vi "_TangoGroupWriteAttribute.vi"(1 "error in":errorcluster, 2 "values":T1(array[cluster]), 3 "attribute name":string, 4 "group id":i32) -> (0 "error out":errorcluster)   [LabVIEW 2014, in "tango.lvlib"]
uses:
  tango.lvlib
  tango_binding.so
panel:
  # "*** READ-ME ***\n\nThis Vi can only write one atrribute at a time on the specified Tango group.\n\nThe attribute value must be speciifed for each device in the group using the \n\"values\" array. The size of \"values\" array must equal the number of devices in the group (an error will occurred otherwise).\n\nThe attribute to write on the group is the one specified by the \"attribute name\" input terminal. Both 'values[i].device-name' and 'values[i].attribute-name' are ignored."
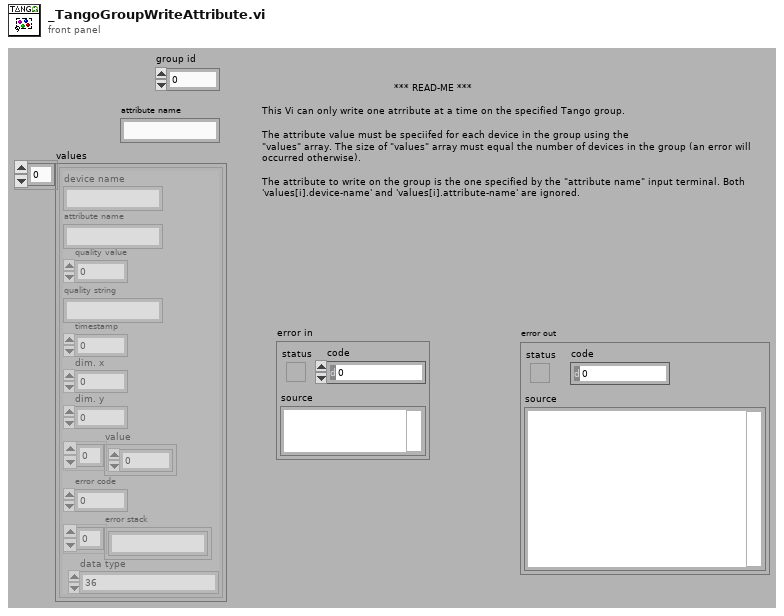
[diagram p1: front panel]
types:
  T1 = cluster{"device name":string, "attribute name":string, "quality value":i16, "quality string":string, "timestamp":dbl, "dim. x":i32, "dim. y":i32, "value":u8[], "error code":i32, "error stack":string[], "data type":u16}[]
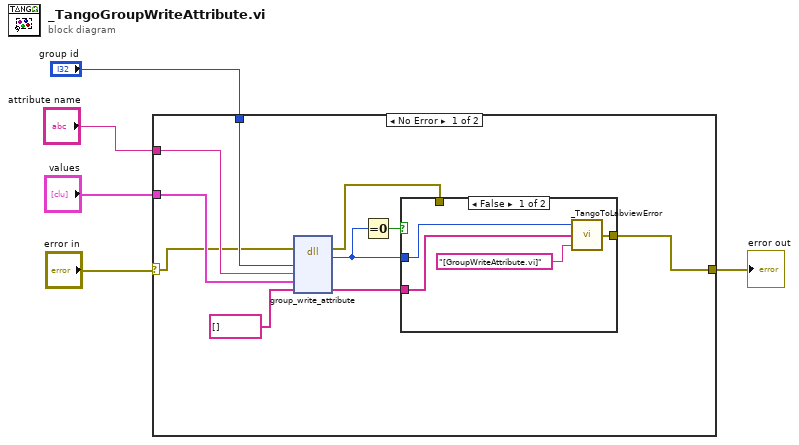
[diagram p0: block diagram]
diagram:
  n1 = case shown="No Error" "error in" {
    selector: "error in" -> [w6 w21]
    tunnel: [w12 w21] -> w4
    tunnel: "values" -> [w10 _]
    tunnel: "attribute name" -> [w9 _]
    tunnel: "group id" -> [w8 _]
    frame No Error {
      n2 = dll-call lib="tango_binding.*" fn="group_write_attribute"(error in=w6, "group_id"=w8, "attribute name"=w9, "attr_values_in"=w10, "error_stack"=string[] [] ("error stack")) -> (error out=w7:errorcluster, "type de retour"=w11:i32, "error_stack"=w13:string[])  [unwired: 5 in, 1 out]
      n3 = Equal To 0?(x=w11) -> (x = 0?=w14:bool)
      n4 = case shown="False" w14 {
        tunnel: [w16 w20] -> w12
        tunnel: w11 -> [w18 _]
        tunnel: w13 -> [w17 _]
        tunnel: w7 -> [_ w20]
        frame False {
          n5 = call "_TangoToLabviewError.vi"("location"="[GroupWriteAttribute.vi]", "error stack"=w17, "error code"=w18) -> ("error out"=w16:errorcluster)
        }
        frame True {
        }
      }
    }
    frame Error {
    }
  }
  "error out" <- w4
